vi "Set CompactSubObj.vi"(8 "error in":errorcluster, 10 "Value":refnum<class "Value.lvclass">, 11 "Object Type in":refnum<class "VAR.lvclass">) -> (0 "error out":errorcluster, 3 "Object Type out":refnum<class "VAR.lvclass">)   [LabVIEW 2024, in "Electronic Datasheet.lvlib" / "VAR.lvclass"]
uses:
  VAR.lvclass
  Value/Value.lvclass
  VAR.lvclass/VAR.ctl
  Electronic Datasheet.lvlib
  D:/git/EDS-File-Viewer/Core/Object Type/Object Type Base.lvclass
  D:/git/EDS-File-Viewer/Core/VAR/VAR.lvclass
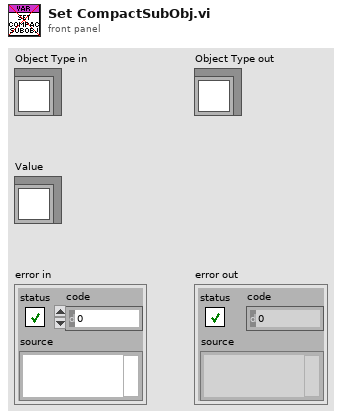
[diagram p1: front panel]
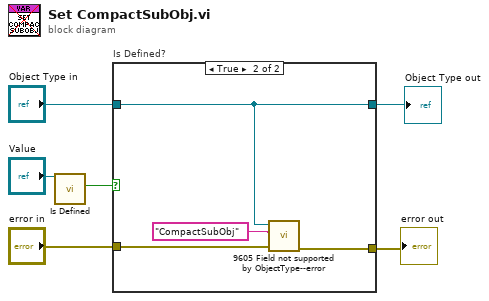
[diagram p0: block diagram]
diagram:
  n1 = call "Is Defined.vi"("Value in"="Value") -> ("Is Defined?"=w5:bool)  [unwired: 9 in, 1 out]
  n2 = case "Is Defined?" shown="True" w5 {
    tunnel: "error in" -> [w8 w11]
    tunnel: "Object Type in" -> [w7 w9]
    tunnel: [w7 w9] -> w2
    tunnel: [w8 w10] -> w1
    frame False {
    }
    frame True {
      n3 = call "9605 Field not supported by ObjectType--error.vi"("error in"=w11, "Field Name"="CompactSubObj" ("Field name"), "Object Type Base"=w9) -> ("error out"=w10:errorcluster)  [unwired: 8 in]
    }
  }
  "error out" <- w1
  "Object Type out" <- w2
